vi "Top and Bottom Stop with Motor.vi"(1 "Bottom DIO":bool, 2 "Motor in":dbl, 3 "Top DIO":bool) -> (0 "Motor out":dbl)   [LabVIEW 2013]
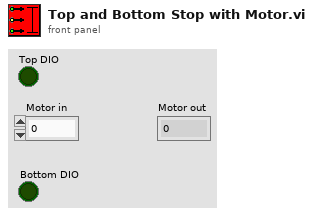
[diagram p1: front panel]
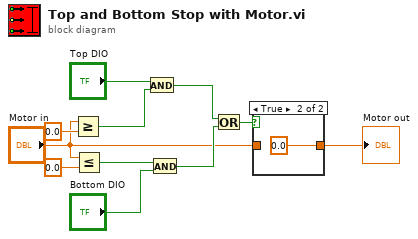
[diagram p0: block diagram]
diagram:
  n1 = Greater Or Equal?(x="Motor in", y=0.0) -> (x >= y?=w8:bool)
  n2 = Less Or Equal?(x="Motor in", y=0.0) -> (x <= y?=w7:bool)
  n3 = And(x="Top DIO", y=w8) -> (x .and. y?=w9:bool)
  n4 = And(x=w7, y="Bottom DIO") -> (x .and. y?=w10:bool)
  n5 = Or(x=w9, y=w10) -> (x .or. y?=w11:bool)
  n6 = case shown="True" w11 {
    tunnel: [w12 0.0 ("axis 2 (y)")] -> w2
    tunnel: "Motor in" -> [w12 _]
    frame False {
    }
    frame True {
    }
  }
  "Motor out" <- w2
